vi "Read A scans.vi"(8 "error in (no error)":errorcluster, 11 "Scan in":refnum<class "Scan.lvclass">) -> (0 "error out":errorcluster, 2 "A scans":dbl=300.0, 3 "Scan out":refnum<class "Scan.lvclass">)   [LabVIEW 2017, in "Scan.lvclass"]
uses:
  Scan.lvclass
  Scan.lvclass/Scan.ctl
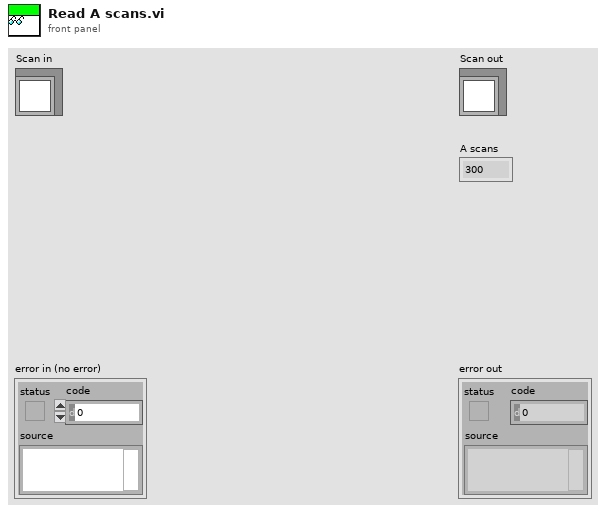
[diagram p1: front panel]
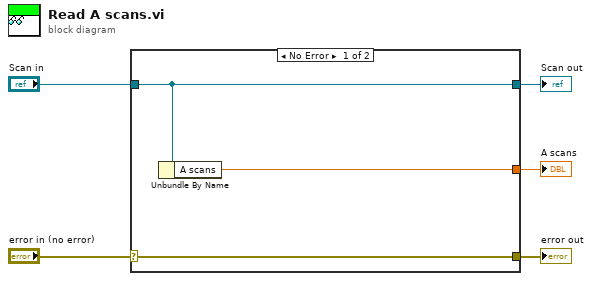
[diagram p0: block diagram]
diagram:
  n1 = case shown="No Error" "error in (no error)" {
    selector: "error in (no error)" -> [w8 w9]
    tunnel: [w8 w9] -> w4
    tunnel: [w7 w10] -> w2
    tunnel: "Scan in" -> [w7 w10]
    tunnel: [w6 _] -> w1
    frame No Error {
      n2 = Unbundle By Name(w7) -> ("A scans"=w6:dbl)
    }
    frame Error {
    }
  }
  "error out" <- w4
  "Scan out" <- w2
  "A scans" <- w1
